vi "Log Event.vi"(8 "error in (no error)":errorcluster caption="错误输入（无错误）", 10 "Event Text":string, 11 "CoordinatorState输入":refnum<class "CoordinatorState.lvclass">) -> (0 "error out":errorcluster caption="错误输出", 3 "Process State out":refnum<class "State Actor.lvclass">)   [LabVIEW 2014, in "States.lvlib" / "CoordinatorState.lvclass"]
uses:
  CoordinatorState.lvclass
  <vilib>/NI/Actors/State Actor/State Actor/State Actor.lvclass
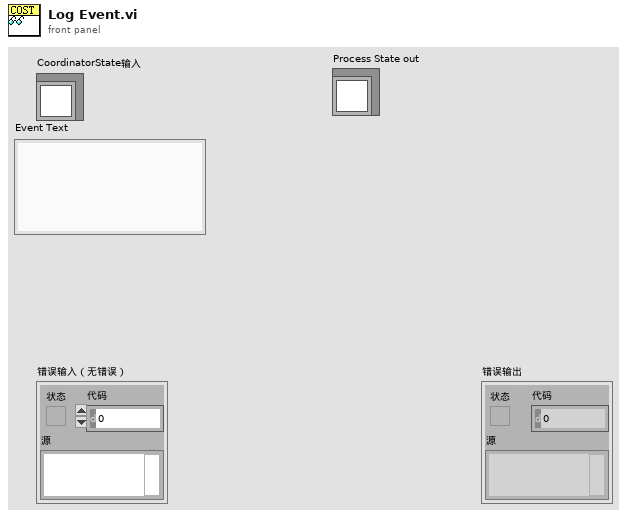
[diagram p1: front panel]
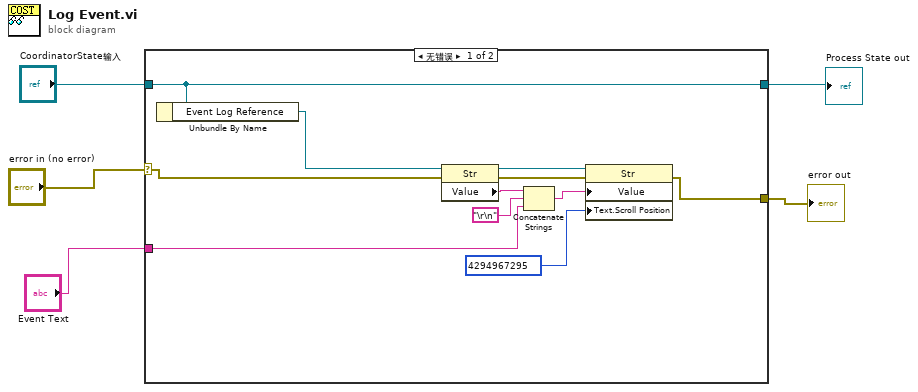
[diagram p0: block diagram]
diagram:
  n1 = case shown="无错误" "error in (no error)" {
    selector: "error in (no error)" -> [w8 w17]
    tunnel: [w6 w17] -> w4
    tunnel: [w16 w18] -> w1
    tunnel: "CoordinatorState输入" -> [w16 w18]
    tunnel: "Event Text" -> [w7 _]
    frame No Error {
      n2 = Unbundle By Name(w16) -> ("Event Log Reference"=w9:refnum<vi>)
      n3 = property class="Str"(reference=w9, error in=w8) -> (reference out=w12:refnum<vi>, error out=w13:errorcluster, "Value"=w10:string)
      n4 = Concatenate Strings(w10, "\r\n", w7) -> (w14:string)
      n5 = property class="Str"(reference=w12, error in=w13, "Value"=w14, "Text.Scroll Position"=u32 4294967295) -> (error out=w6:errorcluster)  [unwired: 1 out]
    }
    frame Error {
    }
  }
  "error out" <- w4
  "Process State out" <- w1
